vi "Update-and-display-module-status.vi"(8 "error in":errorcluster, 10 "Data ref. in":refnum<data-value>, 11 "UI ref. in":refnum<data-value>) -> (0 "error IO":errorcluster, 2 "Data ref.":refnum<data-value>, 3 "UI ref.":refnum<data-value>)   [LabVIEW 2013, in "CameraVision.lvlib" / "CV-UI.lvclass"]
uses:
  CV-UI.lvclass
  Main/CV-Main.lvclass
  Display-names.ctl
  Status-overview.ctl
  Module-states.ctl
  Main/CV-Main.lvclass/CV-Main.ctl
  CV-UI.lvclass/CV-UI.ctl
  Main/Storage/CV-Storage.lvclass/CV-Storage.ctl
  Main/Filter/CV-Filter.lvclass/CV-Filter.ctl
  Main/Mapping/CV-Mapping.lvclass/CV-Mapping.ctl
  Main/Temperature/CV-Temperature.lvclass/CV-Temperature.ctl
  Main/Acquisition/CV-Acquisition.lvclass/CV-Acquisition.ctl
  Main/Configuration/CV-Configuration.lvclass/CV-Configuration.ctl
  Main/Storage/Read Image storage status.vi
  Main/Storage/Read Characteristics storage status.vi
  Main/Storage/Read Temperature storage status.vi
  Main/Storage/Read Storage directory.vi
  Main/Filter/Read Filter status.vi
  Main/Mapping/Read Mapping status.vi
  Main/Temperature/Read Temperature status.vi
  Main/Acquisition/Read Acquisition status.vi
  Main/Acquisition/Read Basic processing status.vi
  Main/Configuration/Read Camera status.vi
  Main/Configuration/Read Grabber status.vi
  Main/Configuration/Read Timing status.vi
  Main/Read Config params.vi
  Main/Read Acquis params.vi
  Main/Read Temperature params.vi
  Main/Read Mapping params.vi
  Main/Read Filter params.vi
  Main/Read Storage params.vi
  Main/Read Processing.vi
  Read Display refs.vi
  Main/Configuration/CV-Configuration.lvclass
  Main/Acquisition/CV-Acquisition.lvclass
  Main/Temperature/CV-Temperature.lvclass
  Main/Mapping/CV-Mapping.lvclass
  Main/Filter/CV-Filter.lvclass
  Main/Storage/CV-Storage.lvclass
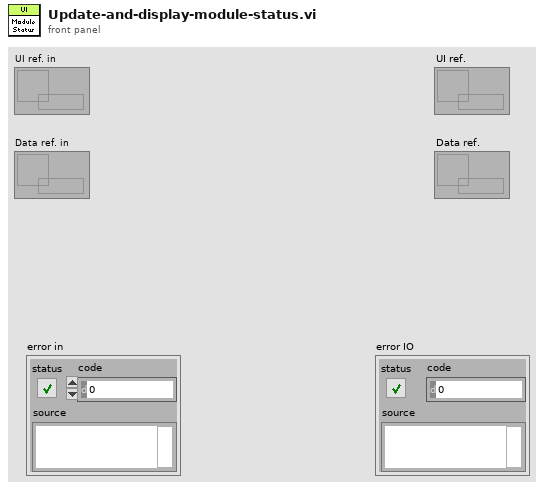
[diagram p1: front panel]
types:
  T1 = typedef "CameraVision.lvlib/CV-UI.lvclass/Display-names.ctl" = enum16{"State", "Action", "Current image", "Framerate", "Frametime", "Process buffer", "Storage buffer", "Free disk space", "Total disk space", "Information", "Histogram", "Camera 1", "Camera 2", "Camera 1 chart", "Camera 2 chart", "Browser", "Temperature", "Map", "Status overview", "Characteristics", "Temper characteristics"}
  T2 = typedef "CameraVision.lvlib/CV-UI.lvclass/Status-overview.ctl" = cluster{"Camera hardware":T3, "Framegrabber":T3, "External timing":T3, "Image acquisition":T3, "Image processing ":T3, "Temperature":T3, "Map":T3, "Storage filter":T3, "Image storage":T3, "Charact. storage":T3, "Temperature storage":T3, "Camera hardware G":bool, "Camera hardware R":bool, "Framegrabber G":bool, "Framegrabber R":bool, "External timing G":bool, "External timing R":bool, "Image acquisition G":bool, "Image acquisition R":bool, "Image processing G":bool, "Image processing R":bool, "Temperature G":bool, "Temperature R":bool, "Map G":bool, "Map R":bool, "Storage filter G":bool, "Storage filter R":bool, "Image storage G":bool, "Image storage R":bool, "Charact storage G":bool, "Charact storage R":bool, "Temperature storage G":bool, "Temperature storage R":bool}
  T3 = typedef "CameraVision.lvlib/CV-UI.lvclass/Module-states.ctl" = enum16{"Inactive", "Active", "Data-loss", "Error", "Simulation", "Synchronizing", "Initialized", "Released"}
  T4 = typedef "Module-status.ctl" = enum16{"Inactive", "Active", "Data-loss", "Error", "Simulation", "Synchronizing", "Initialized", "Released"}
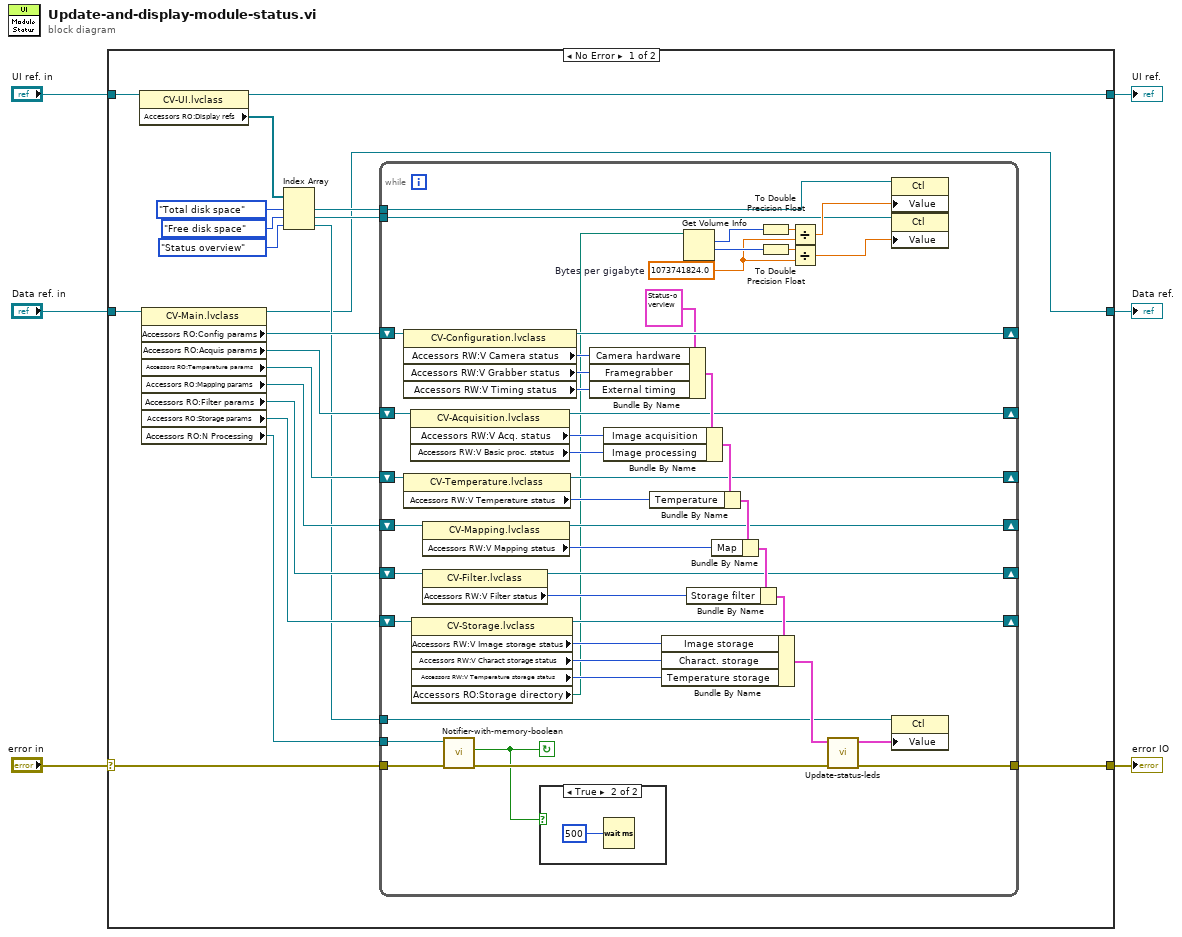
[diagram p0: block diagram]
diagram:
  n1 = case shown="No Error" "error in" {
    selector: "error in" -> [w8 w77]
    tunnel: [w26 w77] -> w6
    tunnel: "UI ref. in" -> [w25 w76]
    tunnel: "Data ref. in" -> [w18 w75]
    tunnel: [w9 w75] -> w2
    tunnel: [w19 w76] -> w1
    frame No Error {
      n2 = property class="CV-UI.lvclass"(reference=w25) -> (reference out=w19:refnum<data-value>, "Accessors RO:Display refs"=w17:refnum<vi>[])  [unwired: 1 in, 1 out]
      n3 = property class="CV-Main.lvclass"(reference=w18) -> (reference out=w9:refnum<data-value>, "Accessors RO:Config params"=w16:refnum<data-value>, "Accessors RO:Acquis params"=w24:refnum<data-value>, "Accessors RO:Temperature params"=w23:refnum<data-value>, "Accessors RO:Mapping params"=w22:refnum<data-value>, "Accessors RO:Filter params"=w21:refnum<data-value>, "Accessors RO:Storage params"=w20:refnum<data-value>, "Accessors RO:N Processing"=w7:refnum<notifier>)  [unwired: 1 in, 1 out]
      n4 = Index Array(array=w17, index #1=Display-names."Total disk space" ("Dislay"), index #2=Display-names."Free disk space" ("Dislay"), index #3=Display-names."Status overview" ("Dislay")) -> (element #1=w12:refnum<vi>, element #2=w11:refnum<vi>, element #3=w10:refnum<vi>)
      n5 = while {
        tunnel: [w28] -> w26
        shift-right: [w46] -> _
        shift-left: w16 -> [w73]
        shift-right: [w47] -> _
        shift-left: w24 -> [w66]
        shift-right: [w48] -> _
        shift-left: w23 -> [w65]
        shift-right: [w49] -> _
        shift-left: w22 -> [w61]
        shift-right: [w50] -> _
        shift-left: w21 -> [w59]
        shift-right: [w51] -> _
        shift-left: w20 -> [w55]
        tunnel: w12 -> [w40]
        tunnel: w11 -> [w35]
        tunnel: w10 -> [w32]
        tunnel: w8 -> [w30]
        tunnel: w7 -> [w31]
        stop <- w27 continue-if-true
        w39 = 1073741824.0  # Bytes per gigabyte
        n6 = property class="CV-Configuration.lvclass"(reference=w73) -> (reference out=w46:refnum<data-value>, "Accessors RW:V Camera status"=w72:T3, "Accessors RW:V Grabber status"=w71:T3, "Accessors RW:V Timing status"=w70:T3)  [unwired: 1 in, 1 out]
        n7 = property class="CV-Temperature.lvclass"(reference=w65) -> (reference out=w48:refnum<data-value>, "Accessors RW:V Temperature status"=w64:T3)  [unwired: 1 in, 1 out]
        n8 = property class="CV-Acquisition.lvclass"(reference=w66) -> (reference out=w47:refnum<data-value>, "Accessors RW:V Acq. status"=w68:T3, "Accessors RW:V Basic proc. status"=w67:T3)  [unwired: 1 in, 1 out]
        n9 = property class="CV-Storage.lvclass"(reference=w55) -> (reference out=w51:refnum<data-value>, "Accessors RW:V Image storage status"=w56:T4, "Accessors RW:V Charact storage status"=w53:T4, "Accessors RW:V Temperature storage status"=w52:T4, "Accessors RO:Storage directory"=w36:path)  [unwired: 1 in, 1 out]
        n10 = property class="CV-Mapping.lvclass"(reference=w61) -> (reference out=w49:refnum<data-value>, "Accessors RW:V Mapping status"=w62:T3)  [unwired: 1 in, 1 out]
        n11 = property class="CV-Filter.lvclass"(reference=w59) -> (reference out=w50:refnum<data-value>, "Accessors RW:V Filter status"=w58:T3)  [unwired: 1 in, 1 out]
        n12 = call "Notifier-with-memory-boolean.vi"("error in"=w30, "Notifier in"=w31) -> ("error IO"=w29:errorcluster, "Notification"=w27:bool)  [unwired: 8 in]
        n13 = case shown="True" w27 {
          frame False {
          }
          frame True {
            n14 = Wait (ms)(milliseconds to wait=u32 500) -> ()  [unwired: 1 out]
          }
        }
        n15 = Bundle By Name(cluster=T2 {"Camera hardware"=enum."Inactive", "Framegrabber"=enum."Inactive", "External timing"=enum."Inactive", "Image acquisition"=enum."Inactive", "Image processing "=enum."Inactive", "Temperature"=enum."Inactive", "Map"=enum."Inactive", "Storage filter"=enum."Inactive", "Image storage"=enum."Inactive", "Charact. storage"=enum."Inactive", "Temperature storage"=enum."Inactive", "Camera hardware G"=FALSE, "Camera hardware R"=FALSE, "Framegrabber G"=FALSE, "Framegrabber R"=FALSE, "External timing G"=FALSE, "External timing R"=FALSE, "Image acquisition G"=FALSE, "Image acquisition R"=FALSE, "Image processing G"=FALSE, "Image processing R"=FALSE, "Temperature G"=FALSE, "Temperature R"=FALSE, "Map G"=FALSE, "Map R"=FALSE, "Storage filter G"=FALSE, "Storage filter R"=FALSE, "Image storage G"=FALSE, "Image storage R"=FALSE, "Charact storage G"=FALSE, "Charact storage R"=FALSE, "Temperature storage G"=FALSE, "Temperature storage R"=FALSE} ("Module status in"), "Camera hardware"=w72, "Framegrabber"=w71, "External timing"=w70) -> (w69:T2)
        n16 = Bundle By Name(cluster=w69, "Image acquisition"=w68, "Image processing"=w67) -> (w63:T2)
        n17 = Bundle By Name(cluster=w63, "Temperature"=w64) -> (w60:T2)
        n18 = Get Volume Info(11:w36) -> (1:w42:i64, 2:w41:i64)  [unwired: 1 in, 4 out]
        n19 = Bundle By Name(cluster=w60, "Map"=w62) -> (w57:T2)
        n20 = Bundle By Name(cluster=w57, "Storage filter"=w58) -> (w54:T2)
        n21 = Bundle By Name(cluster=w54, "Image storage"=w56, "Charact. storage"=w53, "Temperature storage"=w52) -> (w33:T2)
        n22 = To Double Precision Float(number=w41) -> (double precision float=w44:dbl)
        n23 = To Double Precision Float(number=w42) -> (double precision float=w43:dbl)
        n24 = Divide(x=w44, y=w39) -> (x/y=w38:dbl)
        n25 = Divide(x=w43, y=w39) -> (x/y=w37:dbl)
        n26 = call "Update-status-leds.vi"("error in (no error)"=w29, "Module status in"=w33) -> ("error out"=w28:errorcluster, "Module status"=w45:T2)  [unwired: 8 in]
        n27 = property class="Ctl"(reference=w40, "Value"=w38) -> ()  [unwired: 1 in, 2 out]
        n28 = property class="Ctl"(reference=w35, "Value"=w37) -> ()  [unwired: 1 in, 2 out]
        n29 = property class="Ctl"(reference=w32, "Value"=w45) -> ()  [unwired: 1 in, 2 out]
      }
    }
    frame Error {
    }
  }
  "error IO" <- w6
  "Data ref." <- w2
  "UI ref." <- w1
